vi "NFCorpLI5640Lock-inAmp.vi"() -> ()   [LabVIEW 2020]
uses:
  lib/Hardware/TextControlledInstrum/TextControlledInstrum.lvlib
  lib/Hardware/TextControlledInstrum/IOQueuePacket.ctl
  7420c7f9-cfce-4c86-bace-d1ae605820cc.vi
  lib/Hardware/TextControlledInstrum/ControlToCommandMulti.vi
panel:
  in  "Tab Control":enum32{"Setup", "Data"}(tab)=enum."Data"
  in  "Connect":bool
  in  "Serial Port Setting":T1={"stop bits "=10, "flow control (0:none)"=0, "parity (0:none)"=enum."None", "data bits (8)"=8, "termination char for read\n(0xA = '\\n' = LF) "=10, "baud rate"=19200, "LI5640 resource name"="COM7", "timeout (ms)"=200} {"baud rate" items=["110"=110, "300"=300, "600"=600, "1200"=1200, "2400"=2400, "4800"=4800, "9600"=9600, "19200"=19200, "38400"=38400, "57600"=57600, "115200"=115200, "230400"=230400, "460800"=460800, "921600"=921600, "1000000"=1000000, "2000000"=2000000, "4000000"=4000000]; "data bits (8)" min=5 max=8 step=1; "flow control (0:none)" items=["None", "XON/XOFF", "RTS/CTS", "XON/XOFF & RTS/CTS", "DTR/DSR", "XON/XOFF & DTR/DSR"]; "stop bits" items=["1.0"=10, "1.5"=15, "2.0"=20]}
  in  "Auto Update":bool
  in  "Auto Phase":bool
  in  "Setting":T2={"PHAS"=-138.78, "FREQ"=590.0, "AMPL"=0.011, "HARM"=1.0, "RSRC"=0, "REDG"=0, "ISRC"=0, "ICPL"=0, "IGND"=0, "ILIN"=1, "IFRQ"=0, "ITHR"=0, "DRSV"=0, "VSEN"=24, "ISEN"=20, "TCON"=9, "SYNC"=1, "SLOP"=0} {"SLOP" items=["6 dB/oct", "12 dB/oct", "18 dB/oct", "24 dB/oct"]; "SYNC" items=["off", "on"]; "TCON" items=["10 us", "30 us", "100 us", "300 us", "1 ms", "3 ms", "10 ms", "30 ms", "100 ms", "300 ms", "1 s", "3 s", "10 s", "30 s", "100 s", "300 s", "1 ks", "3 ks", "10 ks", "30 ks"]; "ISEN" items=["5 fA", "10 fA", "20 fA", "50 fA", "100 fA", "200 fA", "500 fA", "1 pA", "2 pA", "5 pA", "10 pA", "20 pA", "50 pA", "100 pA", "200 pA", "500 pA", "1 nA", "2 nA", "5 nA", "10 nA", "20 nA", "50 nA", "100 nA", "200 nA", "500 nA", "1 uA"]; "VSEN" items=["2 nV", "5 nV", "10 nV", "20 nV", "50 nV", "100 nV", "200 nV", "500 nV", "1 uV", "2 uV", "5 uV", "10 uV", "20 uV", "50 uV", "100 uV", "200 uV", "500 uV", "1 mV", "2 mV", "5 mV", "10 mV", "20 mV", "50 mV", "100 mV", "200 mV", "500 mV", "1 V"]; "DRSV" items=["HIGH", "MEDIUM", "LOW"]; "ITHR" items=["LPF used", "LPF not used"]; "IFRQ" items=["50 Hz", "60 Hz"]; "ILIN" items=["not used", "LINE", "LINE x 2", "LINE & LINE x 2"]; "IGND" items=["Float", "GND"]; "ICPL" items=["AC", "DC"]; "ISRC" items=["A", "A-B", "I(10^6)", "I(10^8)"]; "REDG" items=["SINE POS", "TTL POS", "TTL NEG"]; "RSRC" items=["REF IN", "INT OSC", "SIGNAL"]}
  out "SlideY":ext(slide)=1.199999999999999889e-10 scale=-1.0..1.0
  out "SlideX":ext(slide)=-5.0529999999999995726e-11 scale=-1.0..1.0
  in  "Factor":ext=1e-10 format="%#_6e"
  out "X":dbl=-1.0105999999999999e-11 format="%#_6p"
  out "Y":dbl=2.3999999999999998e-11 format="%#_6p"
  out "SENSE":dbl=0.2 format="%#_6p"
  out "Serial Port":refnum<visa-resource-name>="COM4"
  # "ロックイン本体の設定に合わせる必要がある\n    SHIFT + SPECIAL で 232 を選択\n    SHIFT + BAUD で 19200 を選択\n    SHIFT + PARITY で none 8 を選択（パリティなし 8bit）\n    SHIFT + ADDRESS で dL = L を選択（改行 LF）"
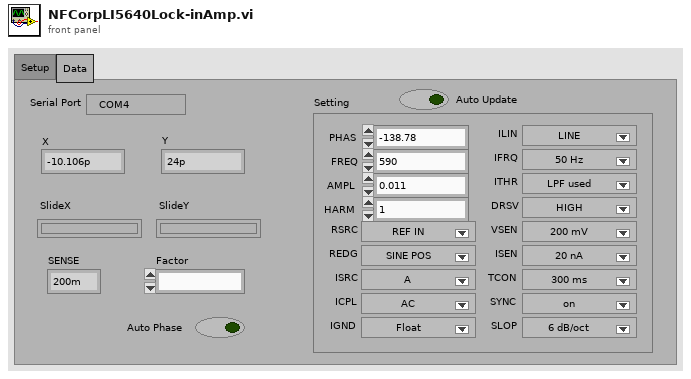
[diagram p1: front panel]
types:
  T1 = cluster{"stop bits ":u16, "flow control (0:none)":u16, "parity (0:none)":enum16{"None", "Odd", "Even", "Mark", "Space"}, "data bits (8)":u16, "termination char for read\n(0xA = '\\n' = LF) ":u8, "baud rate":u32, "LI5640 resource name":refnum<visa-resource-name>, "timeout (ms)":u32}
  T2 = cluster{"PHAS":dbl, "FREQ":dbl, "AMPL":dbl, "HARM":dbl, "RSRC":u16, "REDG":u16, "ISRC":u16, "ICPL":u16, "IGND":u16, "ILIN":u16, "IFRQ":u16, "ITHR":u16, "DRSV":u16, "VSEN":u16, "ISEN":u16, "TCON":u16, "SYNC":u16, "SLOP":u16}
  T3 = typedef "TextControlledInstrum.lvlib/IOQueuePacket.ctl" = cluster{"Operation":enum16{"read", "write", "reserved2", "reserved3", "reserved4", "reserved5", "reserved6", "reserved7"}, "Data":string, "Queue":refnum<queue>}
  T4 = enum16{"read", "write", "reserved2", "reserved3", "reserved4", "reserved5", "reserved6", "reserved7"}
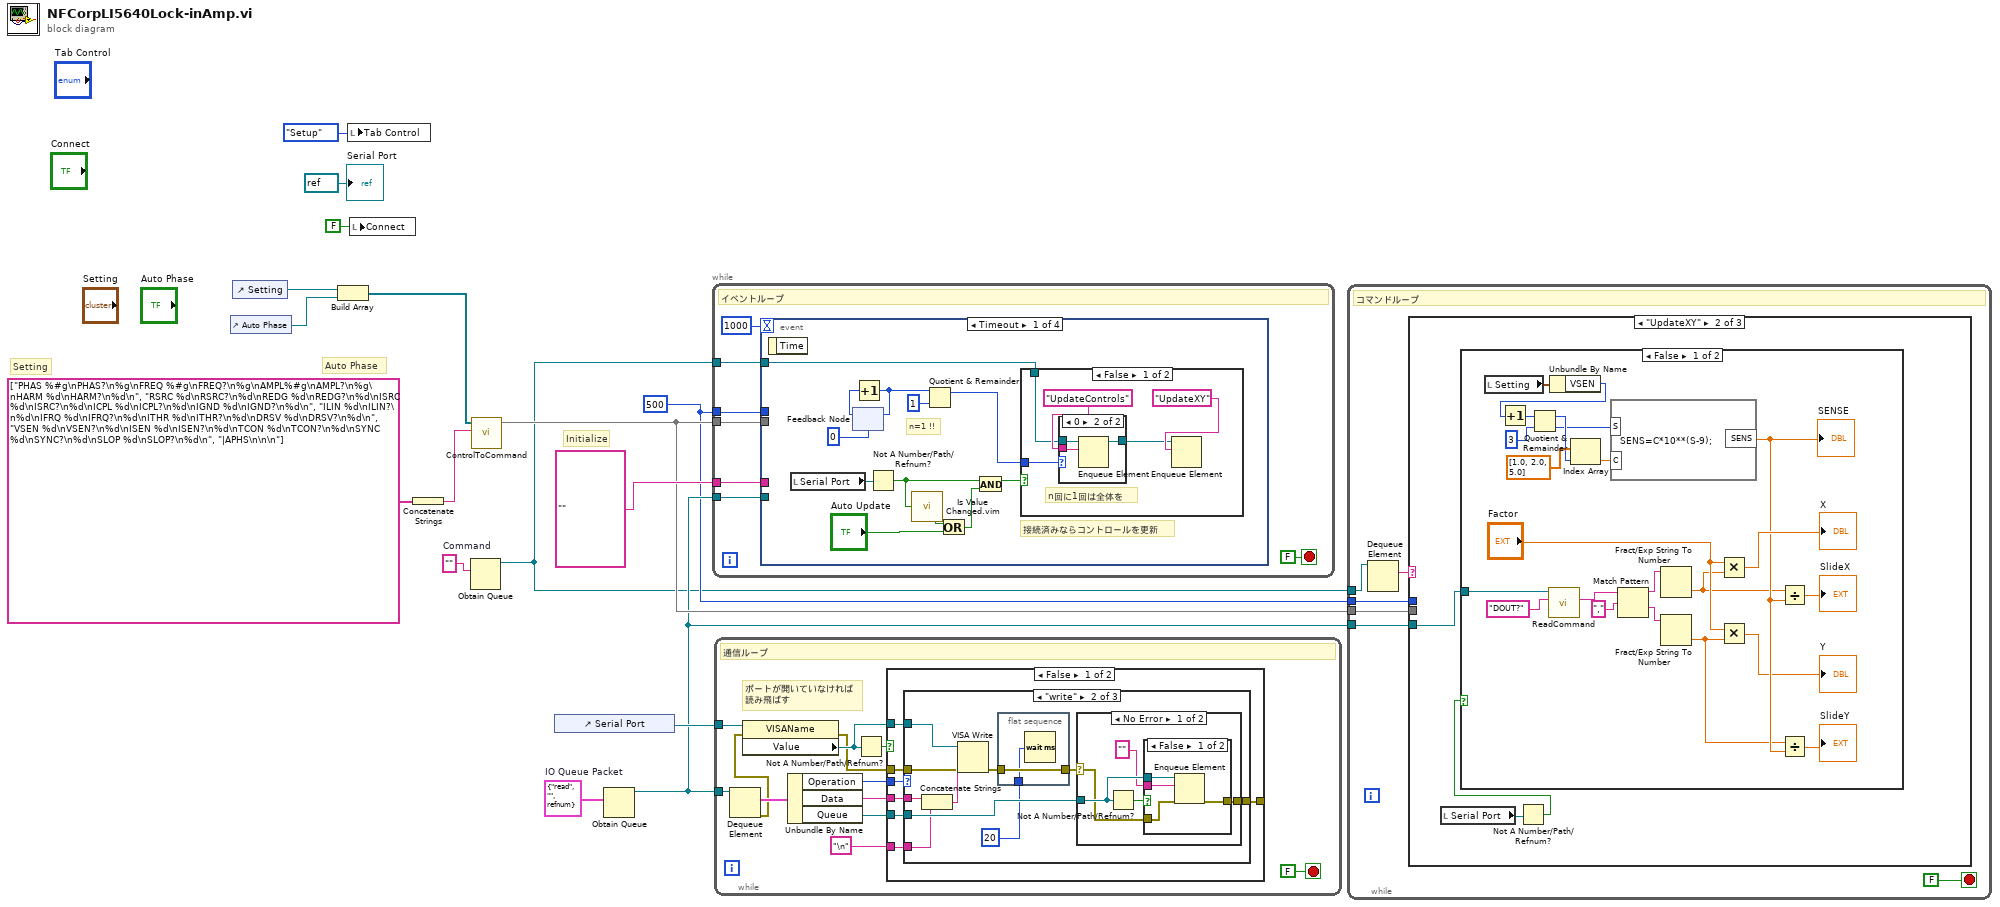
[diagram p0: block diagram]
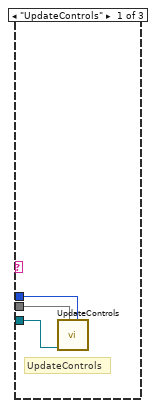
[diagram p2: hidden frame]
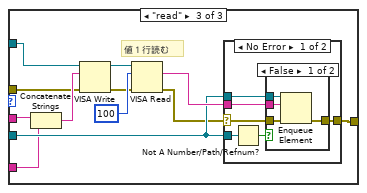
[diagram p8: hidden frame]
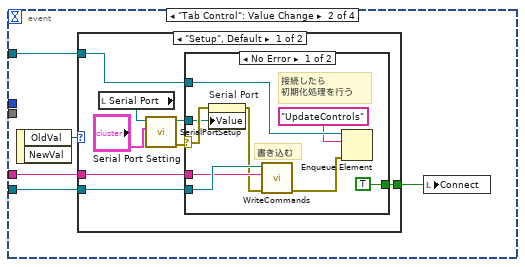
[diagram p14: hidden frame]
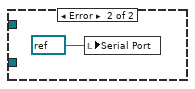
[diagram p15: hidden frame]
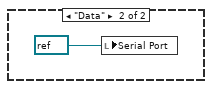
[diagram p16: hidden frame]
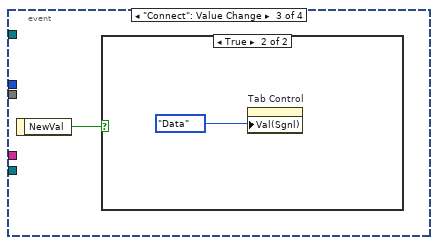
[diagram p17: hidden frame]
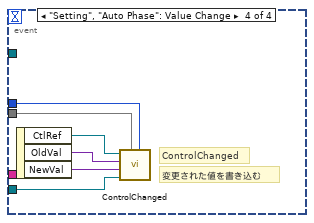
[diagram p19: hidden frame]
diagram:
  w8 = ""  # Command
  w3 = 500 ("timeout")
  w9 = T3 {"Operation"=enum."read", "Data"="", "Queue"=refnum}  # IO Queue Packet
  # "Initialize"
  # "Auto Phase"
  # "Setting"
  n1 = control-ref of="Auto Phase"() -> (w15:refnum<vi>)
  n2 = control-ref of="Setting"() -> (w16:refnum<vi>)
  n3 = Build Array(w16, w15) -> (w14:refnum<vi>[])
  n4 = local write "Tab Control"(enum32{"Setup", "Data"}."Setup" ("Tab Control")) -> ()
  n5 = local write "Connect"(FALSE ("Connect")) -> ()
  n6 = Concatenate Strings(string[] ["PHAS %#g\nPHAS?\n%g\nFREQ %#g\nFREQ?\n%g\nAMPL%#g\nAMPL?\n%g\nHARM %d\nHARM?\n%d\n", "RSRC %d\nRSRC?\n%d\nREDG %d\nREDG?\n%d\nISRC %d\nISRC?\n%d\nICPL %d\nICPL?\n%d\nIGND %d\nIGND?\n%d\n", "ILIN %d\nILIN?\n%d\nIFRQ %d\nIFRQ?\n%d\nITHR %d\nITHR?\n%d\nDRSV %d\nDRSV?\n%d\n", "VSEN %d\nVSEN?\n%d\nISEN %d\nISEN?\n%d\nTCON %d\nTCON?\n%d\nSYNC %d\nSYNC?\n%d\nSLOP %d\nSLOP?\n%d\n", "|APHS\n\n\n"]) -> (w12:string)
  n7 = Obtain Queue(element data type=w8) -> (queue out=w2:refnum<queue>)  [unwired: 4 in, 2 out]
  n8 = call-poly "ControlToCommand.vi"("SetGetCommands"=w12, "Control Array"=w14) -> ("ControlToCommand"=w5:map{refnum<vi>, string[]})  [unwired: 9 in]
  n9 = control-ref of="Serial Port"() -> (w6:refnum<vi>)
  n10 = Obtain Queue(element data type=w9) -> (queue out=w4:refnum<queue>)  [unwired: 4 in, 2 out]
  n11 = while {
    tunnel: w5 -> [w21]
    tunnel: w4 -> [w20]
    tunnel: w3 -> [w19]
    tunnel: w2 -> [w18]
    tunnel: "" -> [w17]
    stop <- FALSE stop-if-true
    # "イベントループ"
    n12 = event shown="[0] Timeout" {
      selector: _ -> [_ _ _ _]
      dyn-events: _ -> [_ _ _ _]
      timeout: 1000 -> [_ _ _ _]
      tunnel: w21 -> [_ _ _ w71]
      tunnel: w20 -> [_ w48 _ w72]
      tunnel: w19 -> [_ _ _ w73]
      tunnel: w18 -> [w35 w47 _ _]
      tunnel: w17 -> [_ w46 _ _]
      event Timeout {
        # "n=1 !!"
        # "接続済みならコントロールを更新"
        n13 = event-data() -> ()  [unwired: 1 in, 1 out]
        n14 = local read "Serial Port"() -> (w34:refnum<visa-resource-name>)
        n15 = feedback #1(0) -> (w27:i32)
        n16 = Increment(x=w27) -> (x+1=w25:i32)
        n17 = feedback-in #1(w25) -> ()
        n18 = Not A Number/Path/Refnum?(number/path/refnum=w34) -> (NaN/Path/Refnum?=w33:bool)
        n19 = call "Is Value Changed.vim"("value"=w33) -> ("changed or first call?"=w31:bool)
        n20 = Quotient & Remainder(x=w25, y=1) -> (x-y*floor(x/y)=w24:i32)  [unwired: 1 out]
        n21 = Or(x=w31, y="Auto Update") -> (x .or. y?=w29:bool)
        n22 = And(x=w33, y=w29) -> (x .and. y?=w30:bool)
        n23 = case shown="False" w30 {
          tunnel: w35 -> [w39 _]
          tunnel: w24 -> [w38 _]
          frame False {
            # "n回に1回は全体を"
            n24 = case shown="0" w38 {
              tunnel: "UpdateControls" -> [_ w44]
              tunnel: w39 -> [w41 w43]
              tunnel: [w41 w42] -> w36
              frame Default {
              }
              frame 0 {
                n25 = Enqueue Element(queue=w43, element=w44) -> (queue out=w42:refnum<queue>)  [unwired: 2 in, 2 out]
              }
            }
            n26 = Enqueue Element(queue=w36, element="UpdateXY") -> ()  [unwired: 2 in, 3 out]
          }
          frame True {
          }
        }
      }
      event "Tab Control": Value Change {
        n27 = event-data() -> ("OldVal"=w49:enum32{"Setup", "Data"})  [unwired: 1 in, 1 out]
        n28 = case shown="\"Setup\", Default" w49 {
          tunnel: w48 -> [w55 _]
          tunnel: w47 -> [w54 _]
          tunnel: w46 -> [w53 _]
          tunnel: [w50 _] -> w45
          frame "Setup", Default {
            n29 = local read "Serial Port"() -> (w57:refnum<visa-resource-name>)
            n30 = call "SerialPortSetup.vi"("Serial Port Setting"="Serial Port Setting", "VISA resource name (will be closed)"=w57) -> ("error out"=w56:errorcluster, "VISA resource name out"=w51:refnum<visa-resource-name>)  [unwired: 8 in]
            n31 = case shown="No Error" w56 {
              selector: w56 -> [w61 _]
              tunnel: w55 -> [w66 _]
              tunnel: w54 -> [w65 _]
              tunnel: w53 -> [w62 _]
              tunnel: w51 -> [w59 _]
              tunnel: [TRUE _] -> w50
              frame No Error {
                # "接続したら\n初期化処理を行う"
                # "書き込む"
                n32 = property on="Serial Port" class="VISAName"(error in=w61, "Value"=w59) -> (error out=w60:errorcluster)  [unwired: 1 in, 1 out]
                n33 = call "WriteCommands.vi"("error in (no error)"=w60, "Multi-line String"=w62, "IO Queue"=w66) -> ("error out"=w63:errorcluster)  [unwired: 7 in, 1 out]
                n34 = Enqueue Element(queue=w65, element="UpdateControls", error in (no error)=w63) -> ()  [unwired: 1 in, 3 out]
              }
              frame Error {
                n35 = local write "Serial Port"(refnum<visa-resource-name> refnum ("t")) -> ()
              }
            }
          }
          frame "Data" {
            n36 = local write "Serial Port"(refnum<visa-resource-name> refnum ("t")) -> ()
          }
        }
        n37 = local write "Connect"(w45) -> ()
      }
      event "Connect": Value Change {
        n38 = event-data() -> ("NewVal"=w69:bool)  [unwired: 1 in]
        n39 = case shown="True" w69 {
          frame False {
          }
          frame True {
            n40 = property on="Tab Control" class="TabCtl (strict)"("Val(Sgnl)"=enum32{"Setup", "Data"}."Data" ("Tab Control")) -> ()  [unwired: 2 in, 2 out]
          }
        }
      }
      event "Setting", "Auto Phase": Value Change {
        # "ControlChanged"
        # "変更された値を書き込む"
        n41 = event-data() -> ("CtlRef"=w76:refnum<vi>, "OldVal"=w75:variant, "NewVal"=w74:variant)  [unwired: 1 in]
        n42 = call "ControlChanged.vi"("timeout in ms (1000ms)"=w73, "ControlToCommand"=w71, "IO Queue"=w72, "NewVal"=w74, "OldVal"=w75, "CtlRef"=w76) -> ()  [unwired: 5 in, 1 out]
      }
    }
  }
  n43 = while {
    tunnel: w4 -> [w86]
    tunnel: w6 -> [w85]
    stop <- FALSE stop-if-true
    # "ポートが開いていなければ\n読み飛ばす"
    # "通信ループ"
    n44 = Dequeue Element(queue=w86) -> (element=w87:T3, error out=w78:errorcluster)  [unwired: 2 in, 2 out]
    n45 = property class="VISAName"(reference=w85, error in=w78) -> (error out=w77:errorcluster, "Value"=w79:refnum<visa-resource-name>)  [unwired: 1 out]
    n46 = Unbundle By Name(w87) -> ("Operation"=w83:T4, "Data"=w81:string, "Queue"=w82:refnum<queue>)
    n47 = Not A Number/Path/Refnum?(number/path/refnum=w79) -> (NaN/Path/Refnum?=w84:bool)
    n48 = case shown="False" w84 {
      tunnel: w83 -> [w95 _]
      tunnel: w79 -> [w94 _]
      tunnel: w81 -> [w93 _]
      tunnel: w82 -> [w92 _]
      tunnel: "\n" -> [w91 _]
      tunnel: w77 -> [w90 w144]
      tunnel: [w89 w144] -> _
      frame False {
        n49 = case shown="\"write\"" w95 {
          tunnel: w94 -> [_ w104 w122]
          tunnel: w93 -> [_ w103 w125]
          tunnel: w92 -> [_ w106 w129]
          tunnel: w91 -> [_ w102 w124]
          tunnel: w90 -> [w96 w100 w121]
          tunnel: [w96 w105 w128] -> w89
          frame Default {
          }
          frame "write" {
            n50 = Concatenate Strings(w103, w102) -> (w101:string)
            n51 = VISA Write(VISA resource name=w104, write buffer=w101, error in (no error)=w100) -> (error out=w99:errorcluster)  [unwired: 2 out]
            n52 = flat-sequence {
              tunnel: w99 -> [w108]
              tunnel: [w108] -> w98
              tunnel: u32 20 ("milliseconds to wait") -> [w107]
              frame #0 {
                n53 = Wait (ms)(milliseconds to wait=w107) -> ()  [unwired: 1 out]
              }
            }
            n54 = case shown="No Error" w98 {
              selector: w98 -> [w109 w119]
              tunnel: w106 -> [w113 _]
              tunnel: [w111 w119] -> w105
              frame No Error {
                n55 = Not A Number/Path/Refnum?(number/path/refnum=w113) -> (NaN/Path/Refnum?=w112:bool)
                n56 = case shown="False" w112 {
                  tunnel: "" -> [w117 _]
                  tunnel: w113 -> [w116 _]
                  tunnel: w109 -> [w115 w118]
                  tunnel: [w114 w118] -> w111
                  frame False {
                    n57 = Enqueue Element(queue=w116, element=w117, error in (no error)=w115) -> (error out=w114:errorcluster)  [unwired: 1 in, 2 out]
                  }
                  frame True {
                  }
                }
              }
              frame Default {
              }
            }
          }
          frame "read" {
            # "値１行読む"
            n58 = Concatenate Strings(w125, w124) -> (w123:string)
            n59 = VISA Write(VISA resource name=w122, write buffer=w123, error in (no error)=w121) -> (VISA resource name out=w127:refnum<visa-resource-name>, error out=w126:errorcluster)  [unwired: 1 out]
            n60 = VISA Read(VISA resource name=w127, byte count=u32 100, error in (no error)=w126) -> (read buffer=w130:string, error out=w120:errorcluster)  [unwired: 2 out]
            n61 = case shown="No Error" w120 {
              selector: w120 -> [w132 w143]
              tunnel: w129 -> [w137 _]
              tunnel: w130 -> [w136 _]
              tunnel: w129 -> [w135 _]
              tunnel: [w133 w143] -> w128
              frame No Error {
                n62 = Not A Number/Path/Refnum?(number/path/refnum=w135) -> (NaN/Path/Refnum?=w134:bool)
                n63 = case shown="False" w134 {
                  tunnel: w137 -> [w141 _]
                  tunnel: w136 -> [w140 _]
                  tunnel: w132 -> [w139 w142]
                  tunnel: [w138 w142] -> w133
                  frame False {
                    n64 = Enqueue Element(queue=w141, element=w140, error in (no error)=w139) -> (error out=w138:errorcluster)  [unwired: 1 in, 2 out]
                  }
                  frame True {
                  }
                }
              }
              frame Default {
              }
            }
          }
        }
      }
      frame True {
      }
    }
  }
  n65 = while {
    tunnel: w5 -> [w148]
    tunnel: w3 -> [w147]
    tunnel: w4 -> [w146]
    tunnel: w2 -> [w145]
    stop <- FALSE stop-if-true
    # "コマンドループ"
    n66 = Dequeue Element(queue=w145) -> (element=w150:string)  [unwired: 2 in, 3 out]
    n67 = case shown="\"UpdateXY\"" w150 {
      tunnel: w147 -> [w153 _ _]
      tunnel: w146 -> [w151 w156 _]
      tunnel: w148 -> [w152 _ _]
      frame "UpdateControls" {
        # "UpdateControls"
        n68 = call "UpdateControls.vi"("timeout in ms (1000ms)"=w153, "ControlToCommand"=w152, "IO Queue"=w151) -> ()  [unwired: 8 in, 1 out]
      }
      frame "UpdateXY" {
        n69 = local read "Serial Port"() -> (w155:refnum<visa-resource-name>)
        n70 = Not A Number/Path/Refnum?(number/path/refnum=w155) -> (NaN/Path/Refnum?=w154:bool)
        n71 = case shown="False" w154 {
          tunnel: w156 -> [w169 _]
          frame False {
            n72 = local read "Setting"() -> (w172:T2)
            n73 = call "ReadCommand.vi"("Command"="DOUT?", "IO Queue"=w169) -> ("Received"=w167:string)  [unwired: 7 in, 2 out]
            n74 = Unbundle By Name(w172) -> ("VSEN"=w171:u16)
            n75 = Increment(x=w171) -> (x+1=w178:u16)
            n76 = Quotient & Remainder(x=w178, y=3) -> (x-y*floor(x/y)=w174:i32, floor(x/y)=w173:i32)
            n77 = Index Array(array=dbl[] [1.0, 2.0, 5.0], index=w174) -> (element=w175:dbl)
            n78 = formula code="SENS=C*10**(S-9);"("S"=w173, "C"=w175) -> ("SENS"=w160:dbl)
            "SENSE" <- w160
            n79 = Match Pattern(string=w167, regular expression=",") -> (before substring=w166:string, after substring=w165:string)  [unwired: 1 in, 2 out]
            n80 = Fract/Exp String To Number(string=w166) -> (number=w157:dbl)  [unwired: 3 in, 1 out]
            n81 = Fract/Exp String To Number(string=w165) -> (number=w158:dbl)  [unwired: 3 in, 1 out]
            n82 = Multiply(x="Factor", y=w157) -> (x*y=→"X":ext)
            n83 = Multiply(x="Factor", y=w158) -> (x*y=→"Y":ext)
            n84 = Divide(x=w157, y=w160) -> (x/y=→"SlideX":dbl)
            n85 = Divide(x=w158, y=w160) -> (x/y=→"SlideY":dbl)
          }
          frame True {
          }
        }
      }
      frame Default {
      }
    }
  }
  "Serial Port" <- refnum<visa-resource-name> refnum ("t")
